vi "DAC Manager New.vi"() -> ()   [LabVIEW 2017]
uses:
  globals/RIO and DAC defaults global.vi
  globals/Global variables.vi
panel:
  out "x-y":u32=25946
  out "size(s)":i32=8
  in  "Correlation array":T1(array[cluster])
  in  "Auto update to evap":bool
  out "ntimes":u32=250001
  out "Output Array":waveform(dbl)[](array[waveform])=[{"t0"=timestamp(0 s since 1904-01-01), "dt"=0.0001, "Y"=array[250002 elements]}, {"t0"=timestamp(0 s since 1904-01-01), "dt"=0.0001, "Y"=array[250002 elements]}, {"t0"=timestamp(0 s since 1904-01-01), "dt"=0.0001, "Y"=array[250002 elements]}, {"t0"=timestamp(0 s since 1904-01-01), "dt"=0.0001, "Y"=array[250002 elements]}, {"t0"=timestamp(0 s since 1904-01-01), "dt"=0.0001, "Y"=array[250002 elements]}, {"t0"=timestamp(0 s since 1904-01-01), "dt"=0.0001, "Y"=array[250002 elements]}, {"t0"=timestamp(0 s since 1904-01-01), "dt"=0.0001, "Y"=array[250002 elements]}, {"t0"=timestamp(0 s since 1904-01-01), "dt"=0.0001, "Y"=array[250002 elements]}]
  out "graph":waveform(dbl)[](graph)=[{"t0"=timestamp(0 s since 1904-01-01), "dt"=0.0001, "Y"=array[250002 elements]}, {"t0"=timestamp(0 s since 1904-01-01), "dt"=0.0001, "Y"=array[250002 elements]}, {"t0"=timestamp(0 s since 1904-01-01), "dt"=0.0001, "Y"=array[250002 elements]}, {"t0"=timestamp(0 s since 1904-01-01), "dt"=0.0001, "Y"=array[250002 elements]}, {"t0"=timestamp(0 s since 1904-01-01), "dt"=0.0001, "Y"=array[250002 elements]}, {"t0"=timestamp(0 s since 1904-01-01), "dt"=0.0001, "Y"=array[250002 elements]}, {"t0"=timestamp(0 s since 1904-01-01), "dt"=0.0001, "Y"=array[250002 elements]}, {"t0"=timestamp(0 s since 1904-01-01), "dt"=0.0001, "Y"=array[250002 elements]}]
  in  "Enable":bool=TRUE
  in  "time step (ms)":dbl=0.1
  in  "DAC Array":T2(array[cluster])=[{"start voltage (V)"="0", "start time (ms)"="0", "Enable DAC"=TRUE, "Hinge points"=[{"time (ms)"="100", "voltage (V)"="5", "transition"=0, "tau"="", "asymptote"="", "end time"=100.0}, {"time (ms)"="200", "voltage (V)"="5", "transition"=1, "tau"="", "asymptote"="", "end time"=200.0}, {"time (ms)"="2000", "voltage (V)"="4", "transition"=0, "tau"="1000", "asymptote"="", "end time"=2000.0}, {"time (ms)"="4000", "voltage (V)"="0.69", "transition"=1, "tau"="120", "asymptote"="1", "end time"=4000.0}, {"time (ms)"="6000", "voltage (V)"="3", "transition"=3, "tau"="250", "asymptote"="1", "end time"=5807.5}, {"time (ms)"="14000", "voltage (V)"="2", "transition"=1, "tau"="", "asymptote"="1", "end time"=14000.0}, {"time (ms)"="", "voltage (V)"="0.069", "transition"=3, "tau"="1000", "asymptote"="1", "end time"=14000.0}, {"time (ms)"="25000", "voltage (V)"="0", "transition"=0, "tau"="", "asymptote"="", "end time"=25000.0}]}, {"start voltage (V)"="0", "start time (ms)"="0", "Enable DAC"=TRUE, "Hinge points"=[{"time (ms)"="100", "voltage (V)"="0", "transition"=0, "tau"="", "asymptote"="", "end time"=100.0}, {"time (ms)"="200", "voltage (V)"="2.5", "transition"=1, "tau"="", "asymptote"="", "end time"=200.0}, {"time (ms)"="12889", "voltage (V)"="2.5", "transition"=0, "tau"="", "asymptote"="", "end time"=12889.0}, {"time (ms)"="13189", "voltage (V)"="1", "transition"=1, "tau"="80", "asymptote"="0.4", "end time"=13189.0}, {"time (ms)"="13289", "voltage (V)"="0.09", "transition"=3, "tau"="250", "asymptote"="1", "end time"=15816.800000000001}, {"time (ms)"="", "voltage (V)"="0.2", "transition"=1, "tau"="", "asymptote"="", "end time"=15816.800000000001}, {"time (ms)"="", "voltage (V)"="0.1", "transition"=3, "tau"="1000", "asymptote"="1", "end time"=15816.800000000001}, {"time (ms)"="25000", "voltage (V)"="0", "transition"=0, "tau"="", "asymptote"="", "end time"=25000.0}]}, {"start voltage (V)"="", "start time (ms)"="", "Enable DAC"=FALSE, "Hinge points"=[{"time (ms)"="100", "voltage (V)"="0", "transition"=0, "tau"="", "asymptote"="", "end time"=100.0}, {"time (ms)"="200", "voltage (V)"="0", "transition"=1, "tau"="", "asymptote"="", "end time"=200.0}, {"time (ms)"="12489", "voltage (V)"="0", "transition"=0, "tau"="", "asymptote"="", "end time"=12489.0}, {"time (ms)"="12789", "voltage (V)"="1.2", "transition"=1, "tau"="", "asymptote"="", "end time"=12789.0}, {"time (ms)"="12889", "voltage (V)"="0.15", "transition"=3, "tau"="150", "asymptote"="1", "end time"=13940.0}, {"time (ms)"="13940", "voltage (V)"="0.15", "transition"=1, "tau"="", "asymptote"="", "end time"=13940.0}, {"time (ms)"="13990", "voltage (V)"="-0.1", "transition"=1, "tau"="", "asymptote"="", "end time"=13990.0}, {"time (ms)"="", "voltage (V)"="", "transition"=0, "tau"="", "asymptote"="", "end time"=13990.0}, {"time (ms)"="15000", "voltage (V)"="0", "transition"=0, "tau"="", "asymptote"="", "end time"=15000.0}]}, {"start voltage (V)"="", "start time (ms)"="", "Enable DAC"=FALSE, "Hinge points"=[]}, {"start voltage (V)"="", "start time (ms)"="", "Enable DAC"=FALSE, "Hinge points"=[]}, {"start voltage (V)"="", "start time (ms)"="", "Enable DAC"=FALSE, "Hinge points"=[]}, {"start voltage (V)"="", "start time (ms)"="", "Enable DAC"=FALSE, "Hinge points"=[]}, {"start voltage (V)"="0", "start time (ms)"="0", "Enable DAC"=FALSE, "Hinge points"=[{"time (ms)"="10", "voltage (V)"="10", "transition"=1, "tau"="", "asymptote"="", "end time"=10.0}, {"time (ms)"="15", "voltage (V)"="0", "transition"=0, "tau"="", "asymptote"="", "end time"=15.0}]}] {"Hinge points"."transition" items=["Step", "Ramp", "Exp", "Bin"]}
  in  "Break":bool
  in  "force channel?":bool[](array[boolean])=[FALSE, FALSE, FALSE, FALSE, FALSE, FALSE, FALSE, FALSE]
  in  "force volts":dbl[](array[numeric])=[0.0, 0.0, 0.0, 1.0, -5.0, 0.0, -0.0, 0.0] format="%.4f"
  in  "Force Out":bool
  in  "Loop":bool=TRUE
  in  "Update":bool
  # "DAC1 Qcoil I   -1 V = 100 A\nDAC2 Qcoil V  6/2  set V = (0.0274 I[A] -0.3)/2.9621\n                             (Vcapacitor=13.6+0.294 I[A]+0.000496 I[A]^2)"
  # "DAC 0            DAC1            DAC 2          DAC 3             DAC4             DAC 5           DAC 6             DAC 7"
  # "EN"
  # "Rel. time"
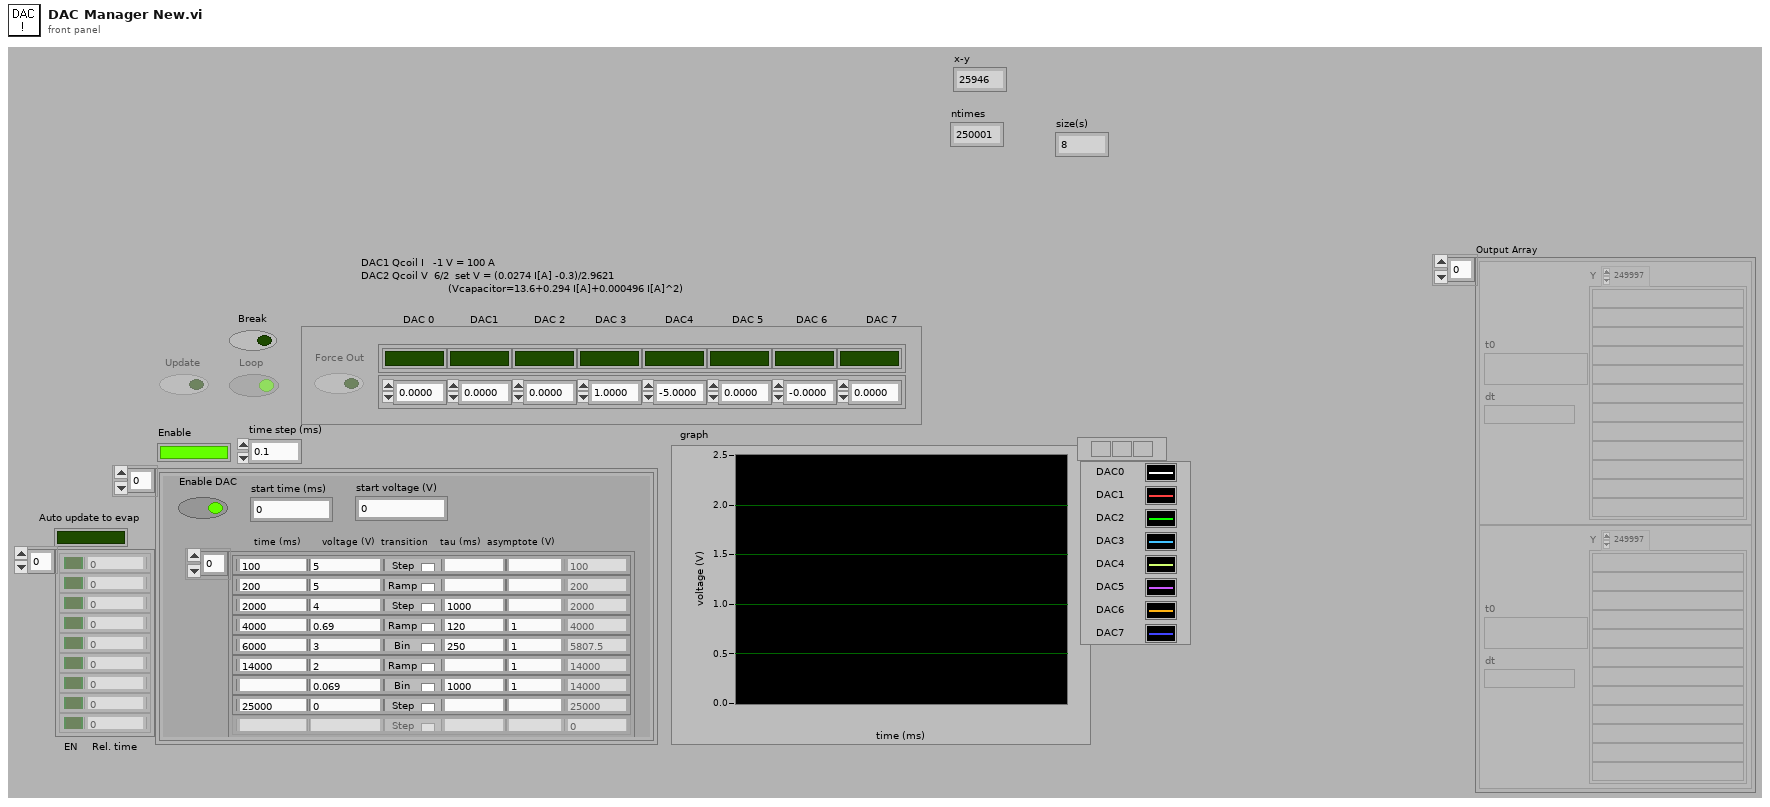
[diagram p1: front panel]
types:
  T1 = cluster{"Correlated to evp ?":bool, "Abs/Rel timing":dbl}[]
  T2 = cluster{"start voltage (V)":string, "start time (ms)":string, "Enable DAC":bool, "Hinge points":cluster{"time (ms)":string, "voltage (V)":string, "transition":u16, "tau":string, "asymptote":string, "end time":dbl}[]}[]
  T3 = enum8{"Enabled", "Disabled", "Disabled and Grayed Out"}
  T4 = cluster{"number":dbl, "number":dbl, "Enable DAC":bool, cluster{"number":dbl, "number":dbl, "transition":u16, "number":dbl, "number":dbl, "end time":dbl}[]}[]
  T5 = cluster{"start voltage (V)":dbl, "start time (ms)":dbl, "Enable DAC":bool, "Hinge points":cluster{"time (ms)":dbl, "voltage (V)":dbl, "transition":u16, "tau":dbl, "asymptote":dbl, "end time":dbl}[]}[]
  T6 = cluster{"time (ms)":string, "voltage (V)":string, "transition":u16, "tau":string}
  T7 = cluster{"start voltage (V)":string, "start time (ms)":string, "Enable DAC":bool, "Hinge points":cluster{"time (ms)":string, "voltage (V)":string, "transition":u16, "tau":string, "asymptote":string, "end time":dbl}[]}
  T8 = cluster{"time (ms)":string, "voltage (V)":string, "transition":u16, "tau":string, "asymptote":string, "end time":dbl}[]
  T9 = cluster{"time (ms)":string, "voltage (V)":string, "transition":u16, "tau":string, "asymptote":string, "end time":dbl}
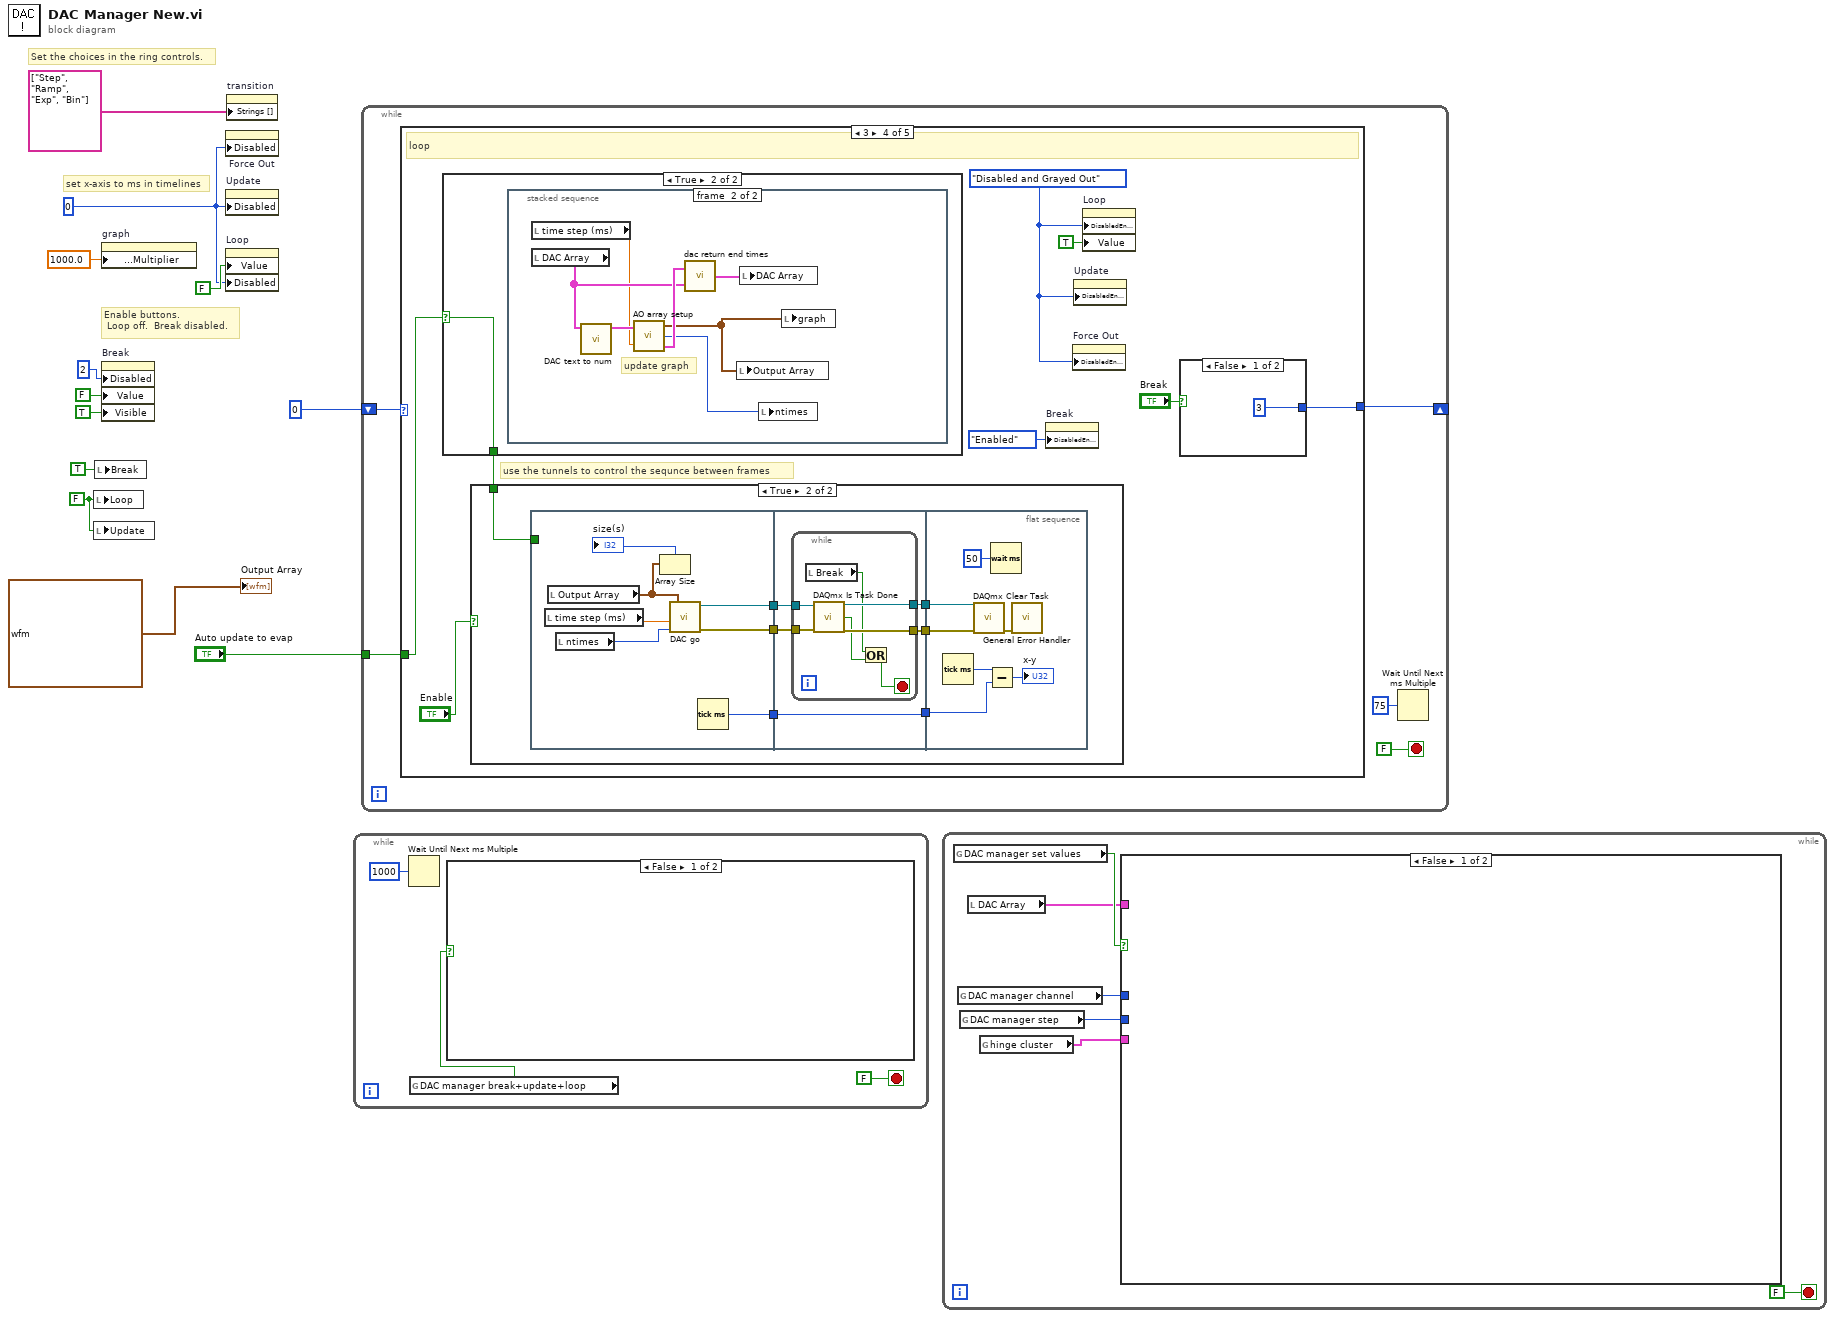
[diagram p0: block diagram]
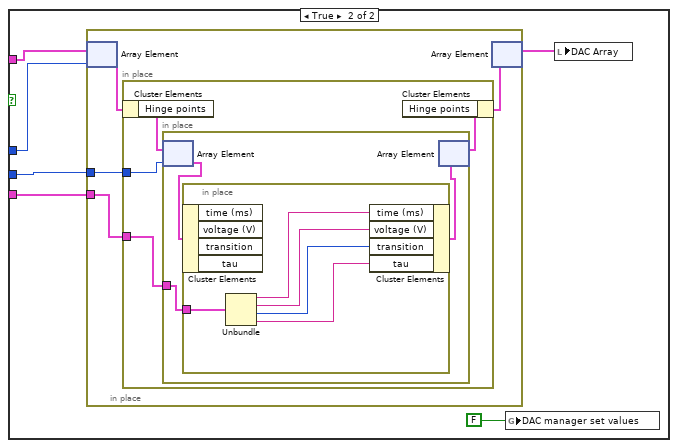
[diagram p2: hidden frame]
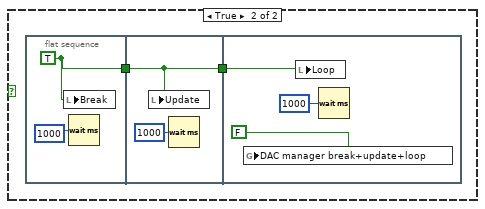
[diagram p3: hidden frame]
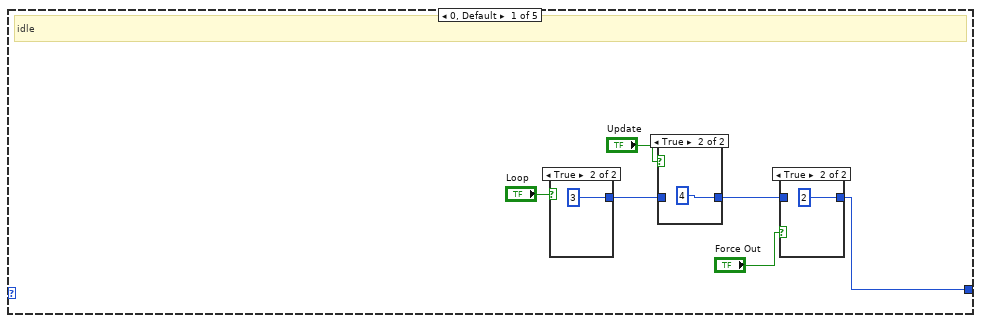
[diagram p4: hidden frame]
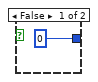
[diagram p7: hidden frame]
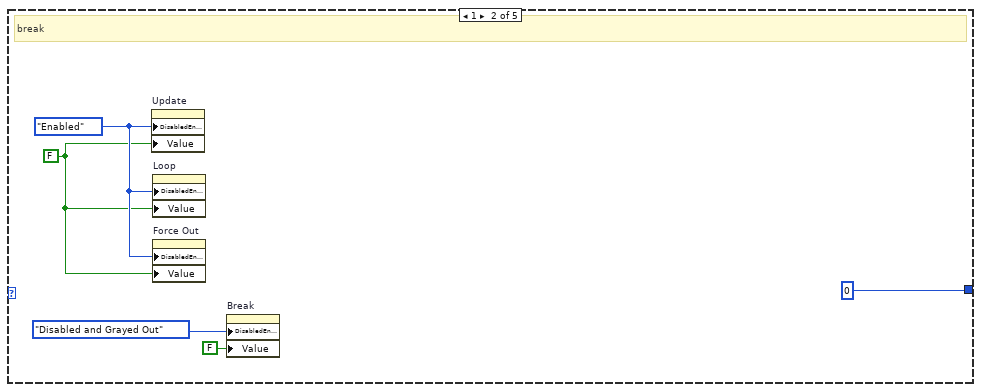
[diagram p8: hidden frame]
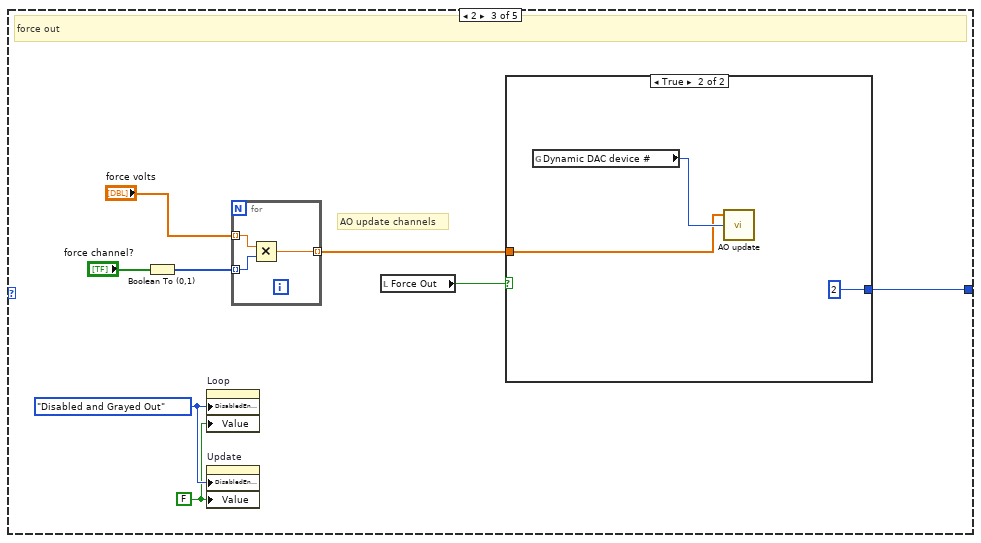
[diagram p9: hidden frame]
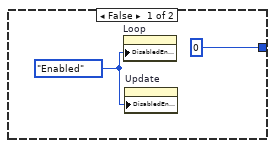
[diagram p10: hidden frame]
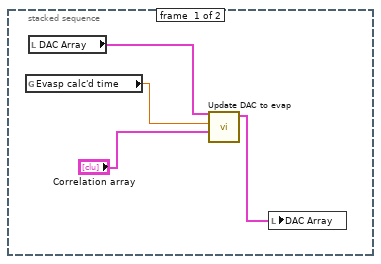
[diagram p12: hidden frame]
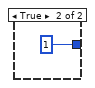
[diagram p14: hidden frame]
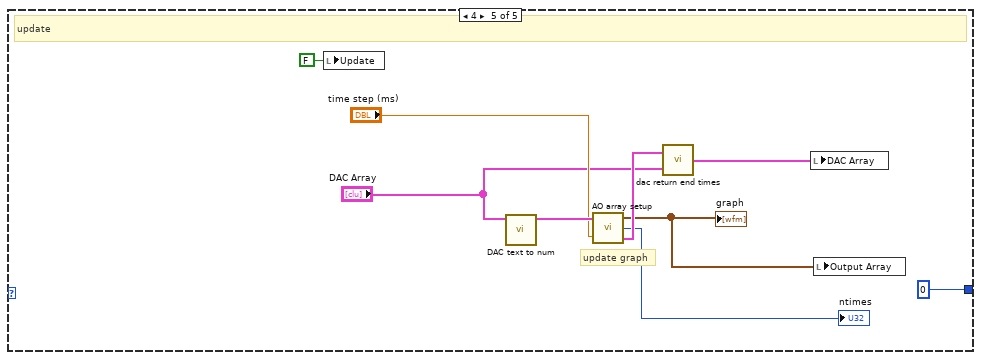
[diagram p15: hidden frame]
diagram:
  w2 = FALSE ("Loop")
  w8 = u8 0 ("Disabled")
  # "set x-axis to ms in timelines"
  # "Enable buttons. \n Loop off.  Break disabled."
  # "Set the choices in the ring controls."
  n1 = local write "Loop"(w2) -> ()
  n2 = local write "Update"(w2) -> ()
  n3 = local write "Break"(TRUE ("Break")) -> ()
  n4 = property on="graph" class="WFGraph (strict)"("X Scale.Offset and Multiplier:Multiplier"=1000.0) -> ()  [unwired: 2 in, 2 out]
  n5 = property on="Break" class="Bool (strict)"("Disabled"=u8 2, "Value"=FALSE ("Break"), "Visible"=TRUE) -> ()  [unwired: 2 in, 2 out]
  n6 = property on="Force Out" class="Bool (strict)"("Disabled"=w8) -> ()  [unwired: 2 in, 2 out]
  n7 = property on="Update" class="Bool (strict)"("Disabled"=w8) -> ()  [unwired: 2 in, 2 out]
  n8 = property on="Loop" class="Bool (strict)"("Value"=FALSE ("Loop"), "Disabled"=w8) -> ()  [unwired: 2 in, 2 out]
  n9 = property on="transition" class="Ring (strict)"("Strings []"=string[] ["Step", "Ramp", "Exp", "Bin"]) -> ()  [unwired: 2 in, 2 out]
  n10 = while {
    stop <- FALSE stop-if-true
    n11 = Wait Until Next ms Multiple(millisecond multiple=u32 1000) -> ()  [unwired: 1 out]
    n12 = global read "Global variables.vi" "DAC manager break+update+loop"() -> (w15:bool)
    n13 = case shown="False" w15 {
      frame False {
      }
      frame True {
        n14 = flat-sequence {
          tunnel: [w19] -> w17
          tunnel: w17 -> [w21]
          tunnel: [w21] -> w16
          tunnel: w16 -> [w24]
          frame #0 {
            w19 = TRUE
            n15 = local write "Break"(w19) -> ()
            n16 = Wait (ms)(milliseconds to wait=u32 1000) -> ()  [unwired: 1 out]
          }
          frame #1 {
            n17 = local write "Update"(w21) -> ()
            n18 = Wait (ms)(milliseconds to wait=u32 1000) -> ()  [unwired: 1 out]
          }
          frame #2 {
            n19 = global write "Global variables.vi" "DAC manager break+update+loop"(FALSE) -> ()
            n20 = local write "Loop"(w24) -> ()
            n21 = Wait (ms)(milliseconds to wait=u32 1000) -> ()  [unwired: 1 out]
          }
        }
      }
    }
  }
  n22 = while {
    shift-right: [w28] -> _
    shift-left: 0 -> [w29]
    tunnel: "Auto update to evap" -> [w25]
    stop <- FALSE stop-if-true
    n23 = case shown="3" w29 {
      tunnel: [w31 0 w54 w68 0] -> w28
      tunnel: w25 -> [_ _ _ w64 _]
      frame 0, Default {
        # "idle"
        n24 = case shown="True" "Loop" {
          tunnel: [0 3] -> w33
          frame False {
          }
          frame True {
          }
        }
        n25 = case shown="True" "Update" {
          tunnel: w33 -> [w38 _]
          tunnel: [w38 4] -> w30
          frame False {
          }
          frame True {
          }
        }
        n26 = case shown="True" "Force Out" {
          tunnel: [w36 2] -> w31
          tunnel: w30 -> [w36 _]
          frame False {
          }
          frame True {
          }
        }
      }
      frame 1 {
        w43 = FALSE ("Update")
        w45 = T3."Enabled" ("Disabled")
        # "break"
        n27 = property on="Update" class="Bool (strict)"("DisabledEnum"=w45, "Value"=w43) -> ()  [unwired: 2 in, 2 out]
        n28 = property on="Loop" class="Bool (strict)"("DisabledEnum"=w45, "Value"=w43) -> ()  [unwired: 2 in, 2 out]
        n29 = property on="Force Out" class="Bool (strict)"("DisabledEnum"=w45, "Value"=w43) -> ()  [unwired: 2 in, 2 out]
        n30 = property on="Break" class="Bool (strict)"("DisabledEnum"=T3."Disabled and Grayed Out" ("Disabled"), "Value"=FALSE ("Break")) -> ()  [unwired: 2 in, 2 out]
      }
      frame 2 {
        w50 = T3."Disabled and Grayed Out" ("Disabled")
        w49 = FALSE ("Loop")
        # "AO update channels"
        # "force out"
        n31 = Boolean To (0,1)(Boolean="force channel?") -> (0, 1=w52:i16[])
        n32 = property on="Loop" class="Bool (strict)"("DisabledEnum"=w50, "Value"=w49) -> ()  [unwired: 2 in, 2 out]
        n33 = property on="Update" class="Bool (strict)"("DisabledEnum"=w50, "Value"=w49) -> ()  [unwired: 2 in, 2 out]
        n34 = for {
          tunnel: "force volts" -> [w57] mode=indexing
          tunnel: w52 -> [w56] mode=indexing
          tunnel: [w55] -> w48 mode=indexing
          n35 = Multiply(x=w57, y=w56) -> (x*y=w55:dbl)
        }
        n36 = local read "Force Out"() -> (w51:bool)
        n37 = case shown="True" w51 {
          tunnel: [0 2] -> w54
          tunnel: w48 -> [_ w60]
          frame False {
            w58 = T3."Enabled" ("Disabled")
            n38 = property on="Loop" class="Bool (strict)"("DisabledEnum"=w58) -> ()  [unwired: 2 in, 2 out]
            n39 = property on="Update" class="Bool (strict)"("DisabledEnum"=w58) -> ()  [unwired: 2 in, 2 out]
          }
          frame True {
            n40 = global read "RIO and DAC defaults global.vi" "Dynamic DAC device #"() -> (w61:i16)
            n41 = call "AO update.vi"("device"=w61, "data"=w60) -> ()  [unwired: 3 in]
          }
        }
      }
      frame 3 {
        w69 = T3."Disabled and Grayed Out" ("Disabled")
        # "use the tunnels to control the sequnce between frames"
        # "loop"
        n42 = case shown="True" w64 {
          selector: w64 -> [w71 w72]
          tunnel: [w71 w72] -> w63
          frame False {
          }
          frame True {
            n43 = stacked-sequence {
              frame #0 {
                n44 = global read "Global variables.vi" "Evasp calc'd time"() -> (w75:dbl)
                n45 = local read "DAC Array"() -> (w76:T2)
                n46 = call "Update DAC to evap.vi"("Control array"="Correlation array", "Evasp calc'd time"=w75, "In Array"=w76) -> ("Out Array"=w74:T2)  [unwired: 8 in]
                n47 = local write "DAC Array"(w74) -> ()
              }
              frame #1 {
                # "update graph"
                n48 = local read "time step (ms)"() -> (w78:dbl)
                n49 = local read "DAC Array"() -> (w80:T2)
                n50 = call "DAC text to num.vi"("In Array"=w80) -> ("Out Array"=w83:T4)  [unwired: 10 in]
                n51 = call "AO array setup.vi"("DAC Array"=w83, "pre-evap time step (ms)"=w78) -> ("Output Array"=w77:waveform(dbl)[], "ntimes"=w79:u32, "DAC Array out"=w82:T5)
                n52 = call "dac return end times.vi"("Text DAC Array In"=w80, "number DAC Array In"=w82) -> ("Text DAC Array Out"=w81:T2)
                n53 = local write "Output Array"(w77) -> ()
                n54 = local write "DAC Array"(w81) -> ()
                n55 = local write "ntimes"(w79) -> ()
                n56 = local write "graph"(w77) -> ()
              }
            }
          }
        }
        n57 = case shown="True" "Enable" {
          tunnel: w63 -> [_ w90]
          frame False {
          }
          frame True {
            n58 = flat-sequence {
              tunnel: [w97] -> w89
              tunnel: [w96] -> w88
              tunnel: w90 -> [_]
              tunnel: [w91] -> w87
              tunnel: w89 -> [w102]
              tunnel: w88 -> [w101]
              tunnel: [w100] -> w86
              tunnel: [w99] -> w85
              tunnel: [w98] -> w84
              tunnel: w87 -> [w98]
              tunnel: w86 -> [w116]
              tunnel: w85 -> [w115]
              tunnel: w84 -> [w111]
              frame #0 {
                n59 = local read "time step (ms)"() -> (w94:dbl)
                n60 = local read "Output Array"() -> (w93:waveform(dbl)[])
                n61 = local read "ntimes"() -> (w95:u32)
                n62 = Array Size(array=w93) -> (size(s)=→"size(s)":i32)
                n63 = call "DAC go.vi"("ntimes"=w95, "time step"=w94, "Input Array"=w93) -> ("error out"=w96:errorcluster, "task out"=w97:refnum<k21>)  [unwired: 3 in]
                n64 = Tick Count (ms)() -> (millisecond timer value=w91:u32)
              }
              frame #1 {
                n65 = while {
                  tunnel: w102 -> [w109]
                  tunnel: w101 -> [w108]
                  tunnel: [w107] -> w100
                  tunnel: [w106] -> w99
                  stop <- w103 stop-if-true
                  n66 = local read "Break"() -> (w105:bool)
                  n67 = call <vilib>:"DAQmx Is Task Done.vi"("task/channels in"=w109, "error in"=w108) -> ("task out"=w107:refnum<k21>, "task done?"=w104:bool, "error out"=w106:errorcluster)  [unwired: 11 in]
                  n68 = Or(x=w105, y=w104) -> (x .or. y?=w103:bool)
                }
              }
              frame #2 {
                n69 = Tick Count (ms)() -> (millisecond timer value=w112:u32)
                n70 = call <vilib>:"DAQmx Clear Task.vi"("task in"=w116, "error in"=w115) -> ("error out"=w114:errorcluster)  [unwired: 13 in]
                n71 = Subtract(x=w112, y=w111) -> (x-y=→"x-y":u32)
                n72 = Wait (ms)(milliseconds to wait=u32 50) -> ()  [unwired: 1 out]
                n73 = call <vilib>:"General Error Handler.vi"("error in (no error)"=w114) -> ()  [unwired: 10 in, 5 out]
              }
            }
          }
        }
        n74 = property on="Break" class="Bool (strict)"("DisabledEnum"=T3."Enabled" ("Disabled")) -> ()  [unwired: 2 in, 2 out]
        n75 = property on="Force Out" class="Bool (strict)"("DisabledEnum"=w69) -> ()  [unwired: 2 in, 2 out]
        n76 = property on="Update" class="Bool (strict)"("DisabledEnum"=w69) -> ()  [unwired: 2 in, 2 out]
        n77 = property on="Loop" class="Bool (strict)"("DisabledEnum"=w69, "Value"=TRUE ("Loop")) -> ()  [unwired: 2 in, 2 out]
        n78 = case shown="False" "Break" {
          tunnel: [3 1] -> w68
          frame False {
          }
          frame True {
          }
        }
      }
      frame 4 {
        # "update graph"
        # "update"
        n79 = local write "Update"(FALSE ("Update")) -> ()
        n80 = call "DAC text to num.vi"("In Array"="DAC Array") -> ("Out Array"=w125:T4)  [unwired: 10 in]
        n81 = call "AO array setup.vi"("DAC Array"=w125, "pre-evap time step (ms)"="time step (ms)") -> ("Output Array"=w122:waveform(dbl)[], "ntimes"=→"ntimes":u32, "DAC Array out"=w124:T5)
        "graph" <- w122
        n82 = call "dac return end times.vi"("Text DAC Array In"="DAC Array", "number DAC Array In"=w124) -> ("Text DAC Array Out"=w123:T2)
        n83 = local write "DAC Array"(w123) -> ()
        n84 = local write "Output Array"(w122) -> ()
      }
    }
    n85 = Wait Until Next ms Multiple(millisecond multiple=u32 75) -> ()  [unwired: 1 out]
  }
  n86 = while {
    stop <- FALSE stop-if-true
    n87 = global read "Global variables.vi" "DAC manager set values"() -> (w133:bool)
    n88 = global read "Global variables.vi" "DAC manager channel"() -> (w131:u8)
    n89 = global read "Global variables.vi" "DAC manager step"() -> (w130:u8)
    n90 = local read "DAC Array"() -> (w132:T2)
    n91 = global read "Global variables.vi" "hinge cluster"() -> (w129:T6)
    n92 = case shown="False" w133 {
      tunnel: w132 -> [_ w138]
      tunnel: w131 -> [_ w137]
      tunnel: w130 -> [_ w136]
      tunnel: w129 -> [_ w139]
      frame False {
      }
      frame True {
        n93 = in-place {
          in-place-border: w139 -> [w143]
          in-place-border: w136 -> [w141]
          n94 = in-place-array #1(w138, w137) -> (w142:T7)
          n95 = in-place {
            in-place-border: w143 -> [w147]
            in-place-border: w141 -> [w145]
            n96 = in-place-cluster #2(w142) -> ("Hinge points"=w146:T8)
            n97 = in-place {
              in-place-border: w147 -> [w148]
              n98 = in-place-array #3(w146, w145) -> (w150:T9)
              n99 = in-place {
                in-place-border: w148 -> [w155]
                n100 = in-place-cluster #4(w150) -> ()  [unwired: 4 out]
                n101 = Unbundle(w155) -> ("time (ms)"=w154:string, "voltage (V)"=w153:string, "transition"=w152:u16, "tau"=w151:string)
                n102 = in-place-cluster #4("time (ms)"=w154, "voltage (V)"=w153, "transition"=w152, "tau"=w151) -> (w149:T9)
              }
              n103 = in-place-array #3(w149) -> (w144:T8)  [unwired: 1 out]
            }
            n104 = in-place-cluster #2("Hinge points"=w144) -> (w140:T7)
          }
          n105 = in-place-array #1(w140) -> (w135:T2)  [unwired: 1 out]
        }
        n106 = global write "Global variables.vi" "DAC manager set values"(FALSE) -> ()
        n107 = local write "DAC Array"(w135) -> ()
      }
    }
  }
  "Output Array" <- waveform(dbl)[] [{"t0"=timestamp(0 s since 1904-01-01), "dt"=0.0001, "Y"=array[250002 elements]}, {"t0"=timestamp(0 s since 1904-01-01), "dt"=0.0001, "Y"=array[250002 elements]}, {"t0"=timestamp(0 s since 1904-01-01), "dt"=0.0001, "Y"=array[250002 elements]}, {"t0"=timestamp(0 s since 1904-01-01), "dt"=0.0001, "Y"=array[250002 elements]}, {"t0"=timestamp(0 s since 1904-01-01), "dt"=0.0001, "Y"=array[250002 elements]}, {"t0"=timestamp(0 s since 1904-01-01), "dt"=0.0001, "Y"=array[250002 elements]}, {"t0"=timestamp(0 s since 1904-01-01), "dt"=0.0001, "Y"=array[250002 elements]}, {"t0"=timestamp(0 s since 1904-01-01), "dt"=0.0001, "Y"=array[250002 elements]}] ("Output Array")
